vi "U64-Array-to-U8-Array.vi"(11 "U64 [] in":u64[](array[numeric]) format="%.0x") -> (3 "U8 [] out":u8[](array[numeric]) format="%.0x")   [LabVIEW 2018]
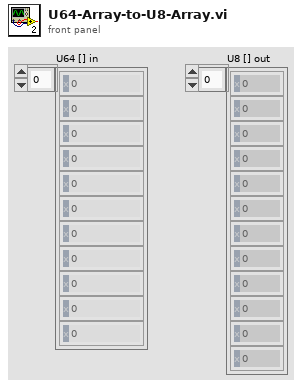
[diagram p1: front panel]
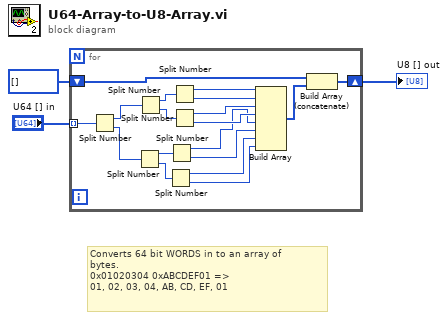
[diagram p0: block diagram]
diagram:
  # "Converts 64 bit WORDS in to an array of\nbytes.\n0x01020304 0xABCDEF01 => \n01, 02, 03, 04, AB, CD, EF, 01"
  n1 = for {
    tunnel: "U64 [] in" -> [w21] mode=indexing
    shift-right: [w17] -> w3
    shift-left: u8[] [] -> [w16]
    n2 = Split Number(x=w21) -> (hi(x)=w20:u32, lo(x)=w19:u32)
    n3 = Split Number(x=w19) -> (hi(x)=w8:u16, lo(x)=w9:u16)
    n4 = Split Number(x=w20) -> (hi(x)=w15:u16, lo(x)=w12:u16)
    n5 = Split Number(x=w9) -> (hi(x)=w6:u8, lo(x)=w7:u8)
    n6 = Split Number(x=w8) -> (hi(x)=w4:u8, lo(x)=w5:u8)
    n7 = Split Number(x=w15) -> (hi(x)=w14:u8, lo(x)=w13:u8)
    n8 = Split Number(x=w12) -> (hi(x)=w10:u8, lo(x)=w11:u8)
    n9 = Build Array(w14, w13, w10, w11, w4, w5, w6, w7) -> (w18:u8[])
    n10 = Build Array (concatenate)(w16, w18) -> (w17:u8[])
  }
  "U8 [] out" <- w3
